vi "XW_Psi_k_wrapper_test_PN.vi"() -> ()   [LabVIEW 2011]
uses:
  Map method.ctl
panel:
  out "Unconverged points (%)":dbl
  out "k2":dbl[](array[numeric])=[0.22919446354040743]
  out "k1":dbl[](array[numeric])=[0.26238974101229007]
  out "Psi2 (deg)":dbl[](array[numeric])=[44.21420620800595]
  out "Psi1 (deg)":dbl[](array[numeric])=[-43.85784811488596]
  out "V (m/s)":dbl[](array[numeric])=[2.943423048907448]
  out "U (m/s)":dbl[](array[numeric])=[7.425777057592518]
  in  "U1cal (m/s)":dbl[](array[numeric])=[10.0]
  in  "U2cal (m/s)":dbl[](array[numeric])=[5.0]
  in  "XW_Calib_Map file path (dialog if empty)":path=path "C:/Documents and Settings/Paul Nathan/Desktop/XW Calib Map/XW angle calib checker/XW_Map_Wire001OH65_080210.txt"
  in  "Map method":T1=enum."Psi_eff, k = f(Umagn.)"
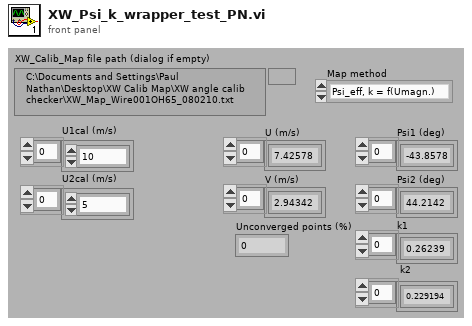
[diagram p1: front panel]
types:
  T1 = typedef "Map method.ctl" = enum16{"Triangle mesh", "Polynomial surface", "Const. Psi_eff (std.)", "Psi_eff = f(Umagn.)", "Psi_eff, k = f(Umagn.)"}
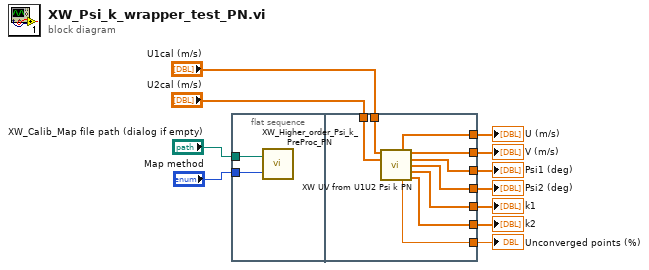
[diagram p0: block diagram]
diagram:
  n1 = flat-sequence {
    tunnel: "Map method" -> [w13]
    tunnel: "XW_Calib_Map file path (dialog if empty)" -> [w12]
    tunnel: "U2cal (m/s)" -> [w22]
    tunnel: "U1cal (m/s)" -> [w21]
    tunnel: [w20] -> w7
    tunnel: [w19] -> w6
    tunnel: [w18] -> w1
    tunnel: [w17] -> w2
    tunnel: [w16] -> w3
    tunnel: [w15] -> w4
    tunnel: [w14] -> w5
    frame #0 {
      n2 = call "XW_Higher_order_Psi_k_PreProc_PN.vi"("Map method"=w13, 2:w12) -> ()  [unwired: 1 out]
    }
    frame #1 {
      n3 = call "XW UV from U1U2 Psi k PN.vi"("U1cal (m/s)"=w21, "U2cal (m/s)"=w22) -> ("U (m/s)"=w20:dbl[], "V (m/s)"=w19:dbl[], "Psi1 (deg)"=w14:dbl[], "Psi2 (deg)"=w15:dbl[], "k1"=w16:dbl[], "Unconverged points (fraction)"=w18:dbl, "k2"=w17:dbl[])  [unwired: 7 out]
    }
  }
  "U (m/s)" <- w7
  "V (m/s)" <- w6
  "Psi1 (deg)" <- w5
  "Psi2 (deg)" <- w4
  "k1" <- w3
  "k2" <- w2
  "Unconverged points (%)" <- w1
